vi "Get_temperature_humidity_from_DB.vi"(0 "log_location":string) -> (1 "log_timestamp":string, 2 "temp_c":string, 3 "rel_hum":string)   [LabVIEW 2021, in "Database Entry.lvclass"]
uses:
  Database Entry.lvclass
  <vilib>/Utility/error.llb/whitespace.ctl
  <vilib>/Utility/file.llb/Read Delimited Spreadsheet (string).vi
panel:
  in  "error in (no error) py":errorcluster
  out "error out py":errorcluster
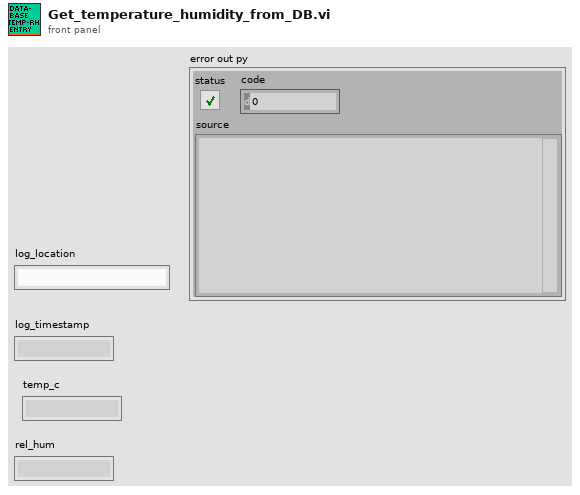
[diagram p1: front panel]
types:
  T1 = typedef "whitespace.ctl" = u16
  T2 = typedef "File Paths.ctl" = cluster{"Glue Pattern Folder":path, "Carrier Tray Folder":path, "Pick Up Tool Fixture Folder":path, "Components Folder":path, "Bellows Tool Offset.txt":path, "Pick Up Tool Offset.txt":path, "Dispense Tip Offset.txt":path, "Log Files":path, "Gantry Assembly Map.txt":path, "Syringe and offset map.txt":path, "Controllers Folder":path, "Local dbase config":path}
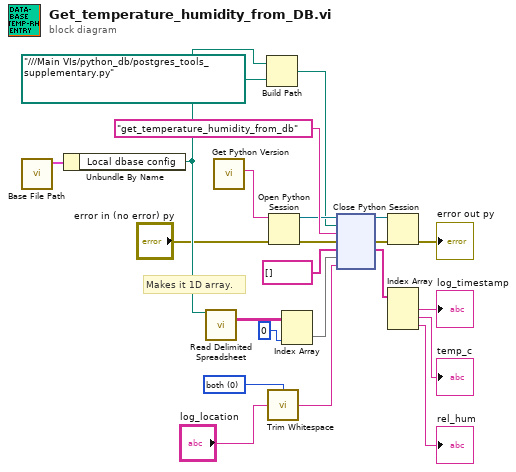
[diagram p0: block diagram]
diagram:
  w1 = T1 0 items=["both", "start of string", "end of string"] ("location (both)")
  # "Makes it 1D array."
  n1 = call "Base File Path.vi"() -> ("Paths Out"=w9:T2)  [unwired: 11 in]
  n2 = Unbundle By Name(w9) -> ("Local dbase config"=w21:path)
  n3 = call-poly <vilib>:"Read Delimited Spreadsheet.vi"("file path (dialog if empty)"=w21) -> ("all rows"=w20:string[][])  [unwired: 9 in, 5 out]
  n4 = call "Get Python Version.vi"() -> ("Python Version"=w19:string)  [unwired: 10 in, 1 out]
  n5 = Build Path(base path=w21, name or relative path=path "../../../Main VIs/python_db/postgres_tools_supplementary.py" ("module path")) -> (appended path=w13:path)
  n6 = call <vilib>:"Trim Whitespace.vi"("string"="log_location", "location (both)"=w1) -> ("trimmed string"=w2:string)
  n7 = Open Python Session(python version=w19, 3:"error in (no error) py") -> (session out=w15:refnum<k35>, error out=w16:errorcluster)  [unwired: 1 in]
  n8 = Index Array(array=w20, index (col)=0 ("disabled index (col)")) -> (element=w12:string[])  [unwired: 1 in]
  n9 = node(w15, w13, "get_temperature_humidity_from_db" ("function name"), w16, string[] [], w12, w2) -> (w11:refnum<k35>, w10:errorcluster, w7:string[])  [unwired: 2 in, 2 out]
  n10 = Close Python Session(session in=w11, error in=w10) -> (11:→"error out py":errorcluster)
  n11 = Index Array(array=w7) -> (element #1=→"log_timestamp":string, element #2=→"temp_c":string, element #3=→"rel_hum":string)  [unwired: 3 in]
